vi "Timer - Cyclical Latch.vi"(7 "Timer (msec)":u32, 11 "Reset (False)":bool) -> (8 "Timer Trigger":bool)   [LabVIEW 2011]
doc: "Points to note about this VI\n\n1) It runs very quickly.\n2) It does not stall the application at this point.\n3) When time passes another unit of the timer, the trigger is set.\n4) The vi must be run in order to trigger. It does not run on an independent thread.\n5) VI is re-entrant. Use as many as you want and they will all be independent."
panel:
  # "Points to note about this VI\n\n1) When time passes another unit of the timer, the trigger is set.\n2) It does not stall the application thread\n3) It runs very quickly.\n4) The vi must be run in order to trigger. It does not run on an independent thread.\n5) VI is re-entrant. Use as many as you want and they will all be independent."
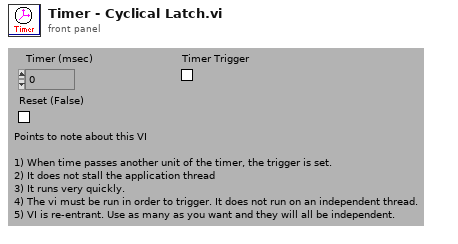
[diagram p1: front panel]
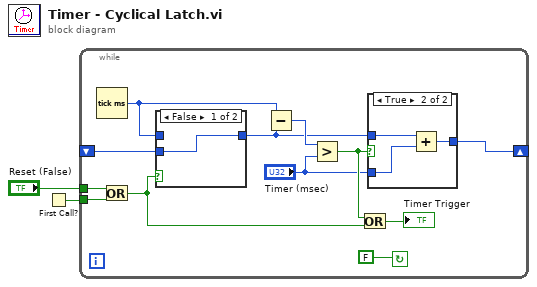
[diagram p0: block diagram]
diagram:
  n1 = First Call?() -> (First Call?: T/F=w2:bool)
  n2 = while {
    shift-right: [w4] -> _
    shift-left: _ -> [w10]
    tunnel: w2 -> [w6]
    tunnel: "Reset (False)" -> [w5]
    stop <- FALSE continue-if-true
    n3 = Tick Count (ms)() -> (millisecond timer value=w9:u32)
    n4 = Or(x=w5, y=w6) -> (x .or. y?=w11:bool)
    n5 = case shown="False" w11 {
      tunnel: w10 -> [w19 _]
      tunnel: w9 -> [_ w20]
      tunnel: [w19 w20] -> w7
      frame False {
      }
      frame True {
      }
    }
    n6 = Subtract(x=w9, y=w7) -> (x-y=w13:u32)
    n7 = Greater?(x=w13, y="Timer (msec)") -> (0:w8:bool)
    n8 = Or(x=w8, y=w11) -> (x .or. y?=→"Timer Trigger":bool)
    n9 = case shown="True" w8 {
      tunnel: w7 -> [w15 w18]
      tunnel: [w15 w17] -> w4
      tunnel: "Timer (msec)" -> [_ w16]
      frame False {
      }
      frame True {
        n10 = Add(x=w18, y=w16) -> (x+y=w17:u32)
      }
    }
  }
